vi "Sandbox 7 - Preview CTL Front Panel.vi"() -> ()   [LabVIEW 2022 SP3]
uses:
  <vilib>/Utility/miscctls.llb/LVPointTypeDef.ctl
  821c8aed-4206-4f88-bf05-8c954f53143e.vi
panel:
  out "error out":errorcluster
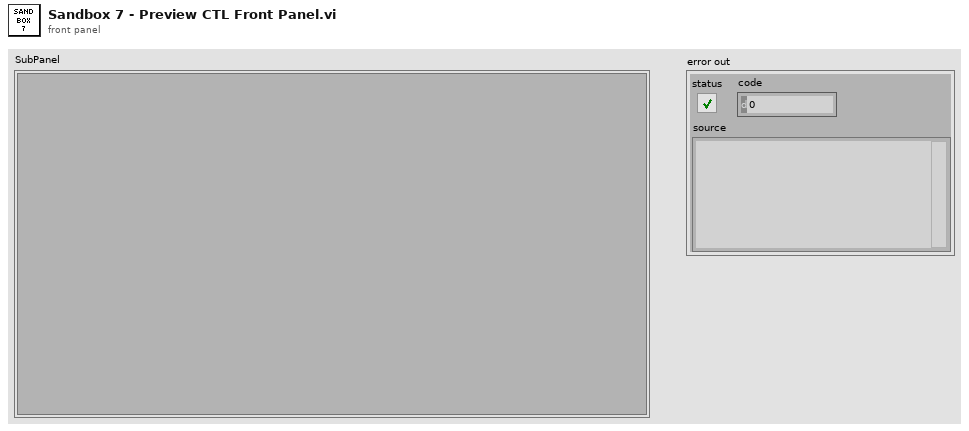
[diagram p1: front panel]
types:
  T1 = typedef "LVPointTypeDef.ctl" = cluster{"Horizontal":i16, "Vertical":i16}
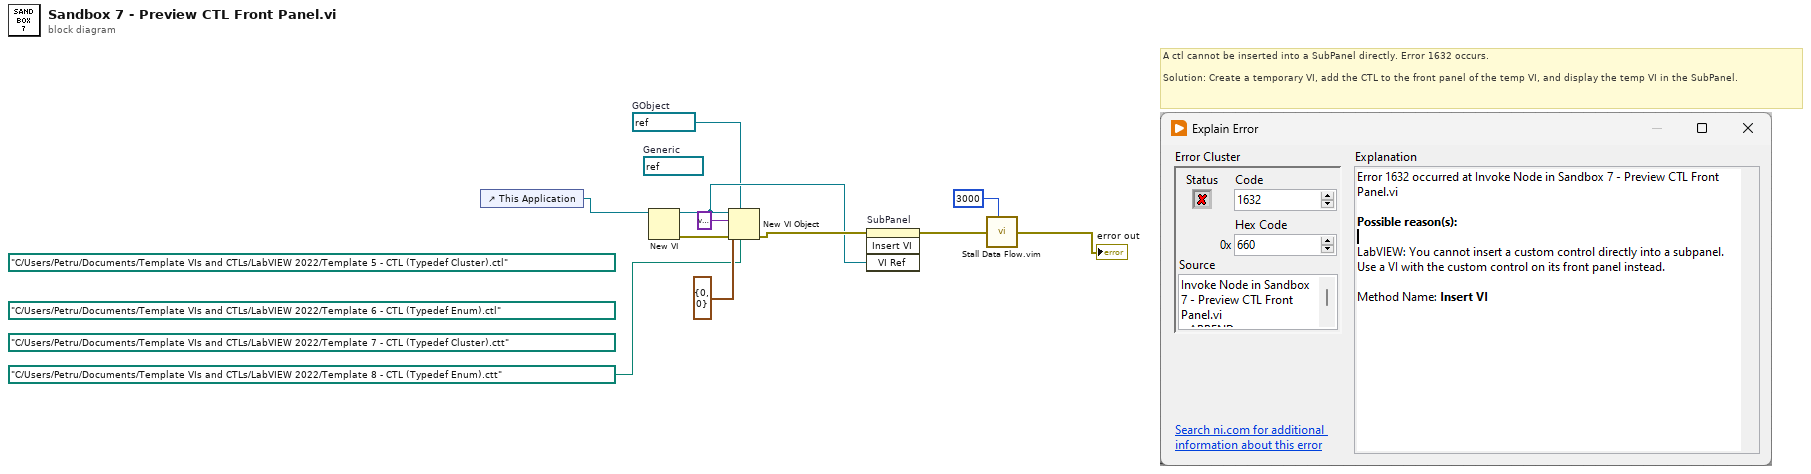
[diagram p0: block diagram]
diagram:
  (unwired) path "C:/Users/Petru/Documents/Template VIs and CTLs/LabVIEW 2022/Template 7 - CTL (Typedef Cluster).ctt"
  w2 = refnum<vi> refnum  # GObject
  (unwired) refnum<vi> refnum  # Generic
  (unwired) path "C:/Users/Petru/Documents/Template VIs and CTLs/LabVIEW 2022/Template 5 - CTL (Typedef Cluster).ctl"
  (unwired) path "C:/Users/Petru/Documents/Template VIs and CTLs/LabVIEW 2022/Template 6 - CTL (Typedef Enum).ctl"
  # "A ctl cannot be inserted into a SubPanel directly. Error 1632 occurs.\n\nSolution: Create a temporary VI, add the CTL to the front panel of the temp VI, and display the temp VI in the SubPanel."
  n1 = control-ref of="This Application"() -> (w10:refnum<vi>)
  n2 = New VI(11:w10) -> (0:w9:errorcluster, 3:w7:refnum<vi>)  [unwired: 6 in]
  n3 = New VI Object(vi object class=w2, owner refnum=w7, style=variant, position/next to=T1 {"Horizontal"=0, "Vertical"=0} ("location"), 6:path "C:/Users/Petru/Documents/Template VIs and CTLs/LabVIEW 2022/Template 8 - CTL (Typedef Enum).ctt", 8:w9) -> (0:w8:errorcluster)  [unwired: 2 in, 1 out]
  n4 = invoke on="SubPanel" class="SubPnl" method="Insert VI"(error in=w8, "VI Ref"=w7) -> (error out=w11:errorcluster)  [unwired: 2 in, 3 out]
  n5 = call "Stall Data Flow.vim"("value in"=w11, "milliseconds to wait"=u32 3000) -> ("value out"=→"error out":errorcluster)  [unwired: 1 out]
